vi "trigVoltages_to_Samples.vi"(10 "resolution (s)":dbl, 11 "Trigger Options":T2={"Trigger Enabled"=FALSE, "Trigger Source"=enum."Channel A", "Trigger Threshold (-5 to 5 V)"=0.0, "Trigger Slope"=2, "Trigger Delay (s)"=0.0, "Auto Trigger Time (ms)"=1000} {"Trigger Delay (s)" min=0.0 format="%#_6f"; "Trigger Slope" items=["Rising"=2, "Falling"=3]; "Trigger Threshold (-5 to 5 V)" format="%#_6p"}) -> (2 "Trigger Settings":T1={"Trigger Enabled"=TRUE, "Trigger Source"=enum."Channel A", "Trigger Threshold (16-bit counts)"=16384, "Trigger Direction"=2, "Trigger Delay (samples)"=0, "Auto Trigger Time (ms)"=0} {"Trigger Direction" items=["Rising"=2, "Falling"=3]})   [LabVIEW 2016]
uses:
  Controls/PicoScope/pico_trigger.ctl
panel:
  in  "Trigger Settings 2":T1={"Trigger Enabled"=TRUE, "Trigger Source"=enum."Channel A", "Trigger Threshold (16-bit counts)"=16384, "Trigger Direction"=2, "Trigger Delay (samples)"=0, "Auto Trigger Time (ms)"=0} {"Trigger Direction" items=["Rising"=2, "Falling"=3]}
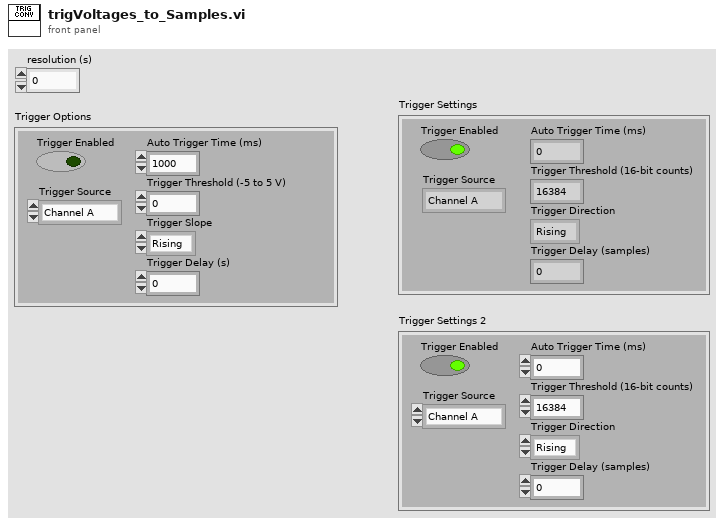
[diagram p1: front panel]
types:
  T1 = cluster{"Trigger Enabled":bool, "Trigger Source":enum16{"Channel A", "Channel B", "Channel C", "Channel D", "Ext."}, "Trigger Threshold (16-bit counts)":i16, "Trigger Direction":u16, "Trigger Delay (samples)":u32, "Auto Trigger Time (ms)":i16}
  T2 = typedef "pico_trigger.ctl" = cluster{"Trigger Enabled":bool, "Trigger Source":enum16{"Channel A", "Channel B", "Channel C", "Channel D", "Ext."}, "Trigger Threshold (-5 to 5 V)":dbl, "Trigger Slope":u16, "Trigger Delay (s)":dbl, "Auto Trigger Time (ms)":i16}
  T3 = enum16{"Channel A", "Channel B", "Channel C", "Channel D", "Ext."}
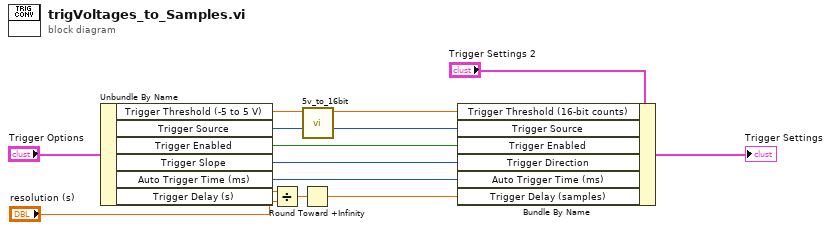
[diagram p0: block diagram]
diagram:
  n1 = Unbundle By Name("Trigger Options") -> ("Trigger Threshold (-5 to 5 V)"=w6:dbl, "Trigger Source"=w9:T3, "Trigger Enabled"=w7:bool, "Trigger Slope"=w10:u16, "Auto Trigger Time (ms)"=w8:i16, "Trigger Delay (s)"=w4:dbl)
  n2 = Divide(x=w4, y="resolution (s)") -> (x/y=w2:dbl)
  n3 = Round Toward +Infinity(x=w2) -> (ceil(x): smallest int >= x=w1:dbl)
  n4 = call "5v_to_16bit.vi"("voltage"=w6) -> ("Bits"=w5:dbl)  [unwired: 10 in]
  n5 = Bundle By Name(cluster="Trigger Settings 2", "Trigger Threshold (16-bit counts)"=w5, "Trigger Source"=w9, "Trigger Enabled"=w7, "Trigger Direction"=w10, "Auto Trigger Time (ms)"=w8, "Trigger Delay (samples)"=w1) -> (→"Trigger Settings":T1)
